vi "Configure Dialog.vi"(8 "error in (no error)":errorcluster, 11 "Configure Trigger Coupling Msg.lvclass":refnum<class "Configure Trigger Coupling Msg.lvclass">) -> (0 "error out":errorcluster, 2 "Ok?":bool, 3 "Configure Trigger Coupling Msg.lvclass":refnum<class "Configure Trigger Coupling Msg.lvclass">)   [LabVIEW 2014, in "CS++Scope.lvlib" / "Configure Trigger Coupling Msg.lvclass"]
uses:
  Configure Trigger Coupling Msg.lvclass
  Configure Trigger Coupling Msg.lvclass/Configure Trigger Coupling Msg.ctl
panel:
  in  "trigger coupling (DC)":i32
  in  "Cancel Button":bool
  in  "OK Button":bool
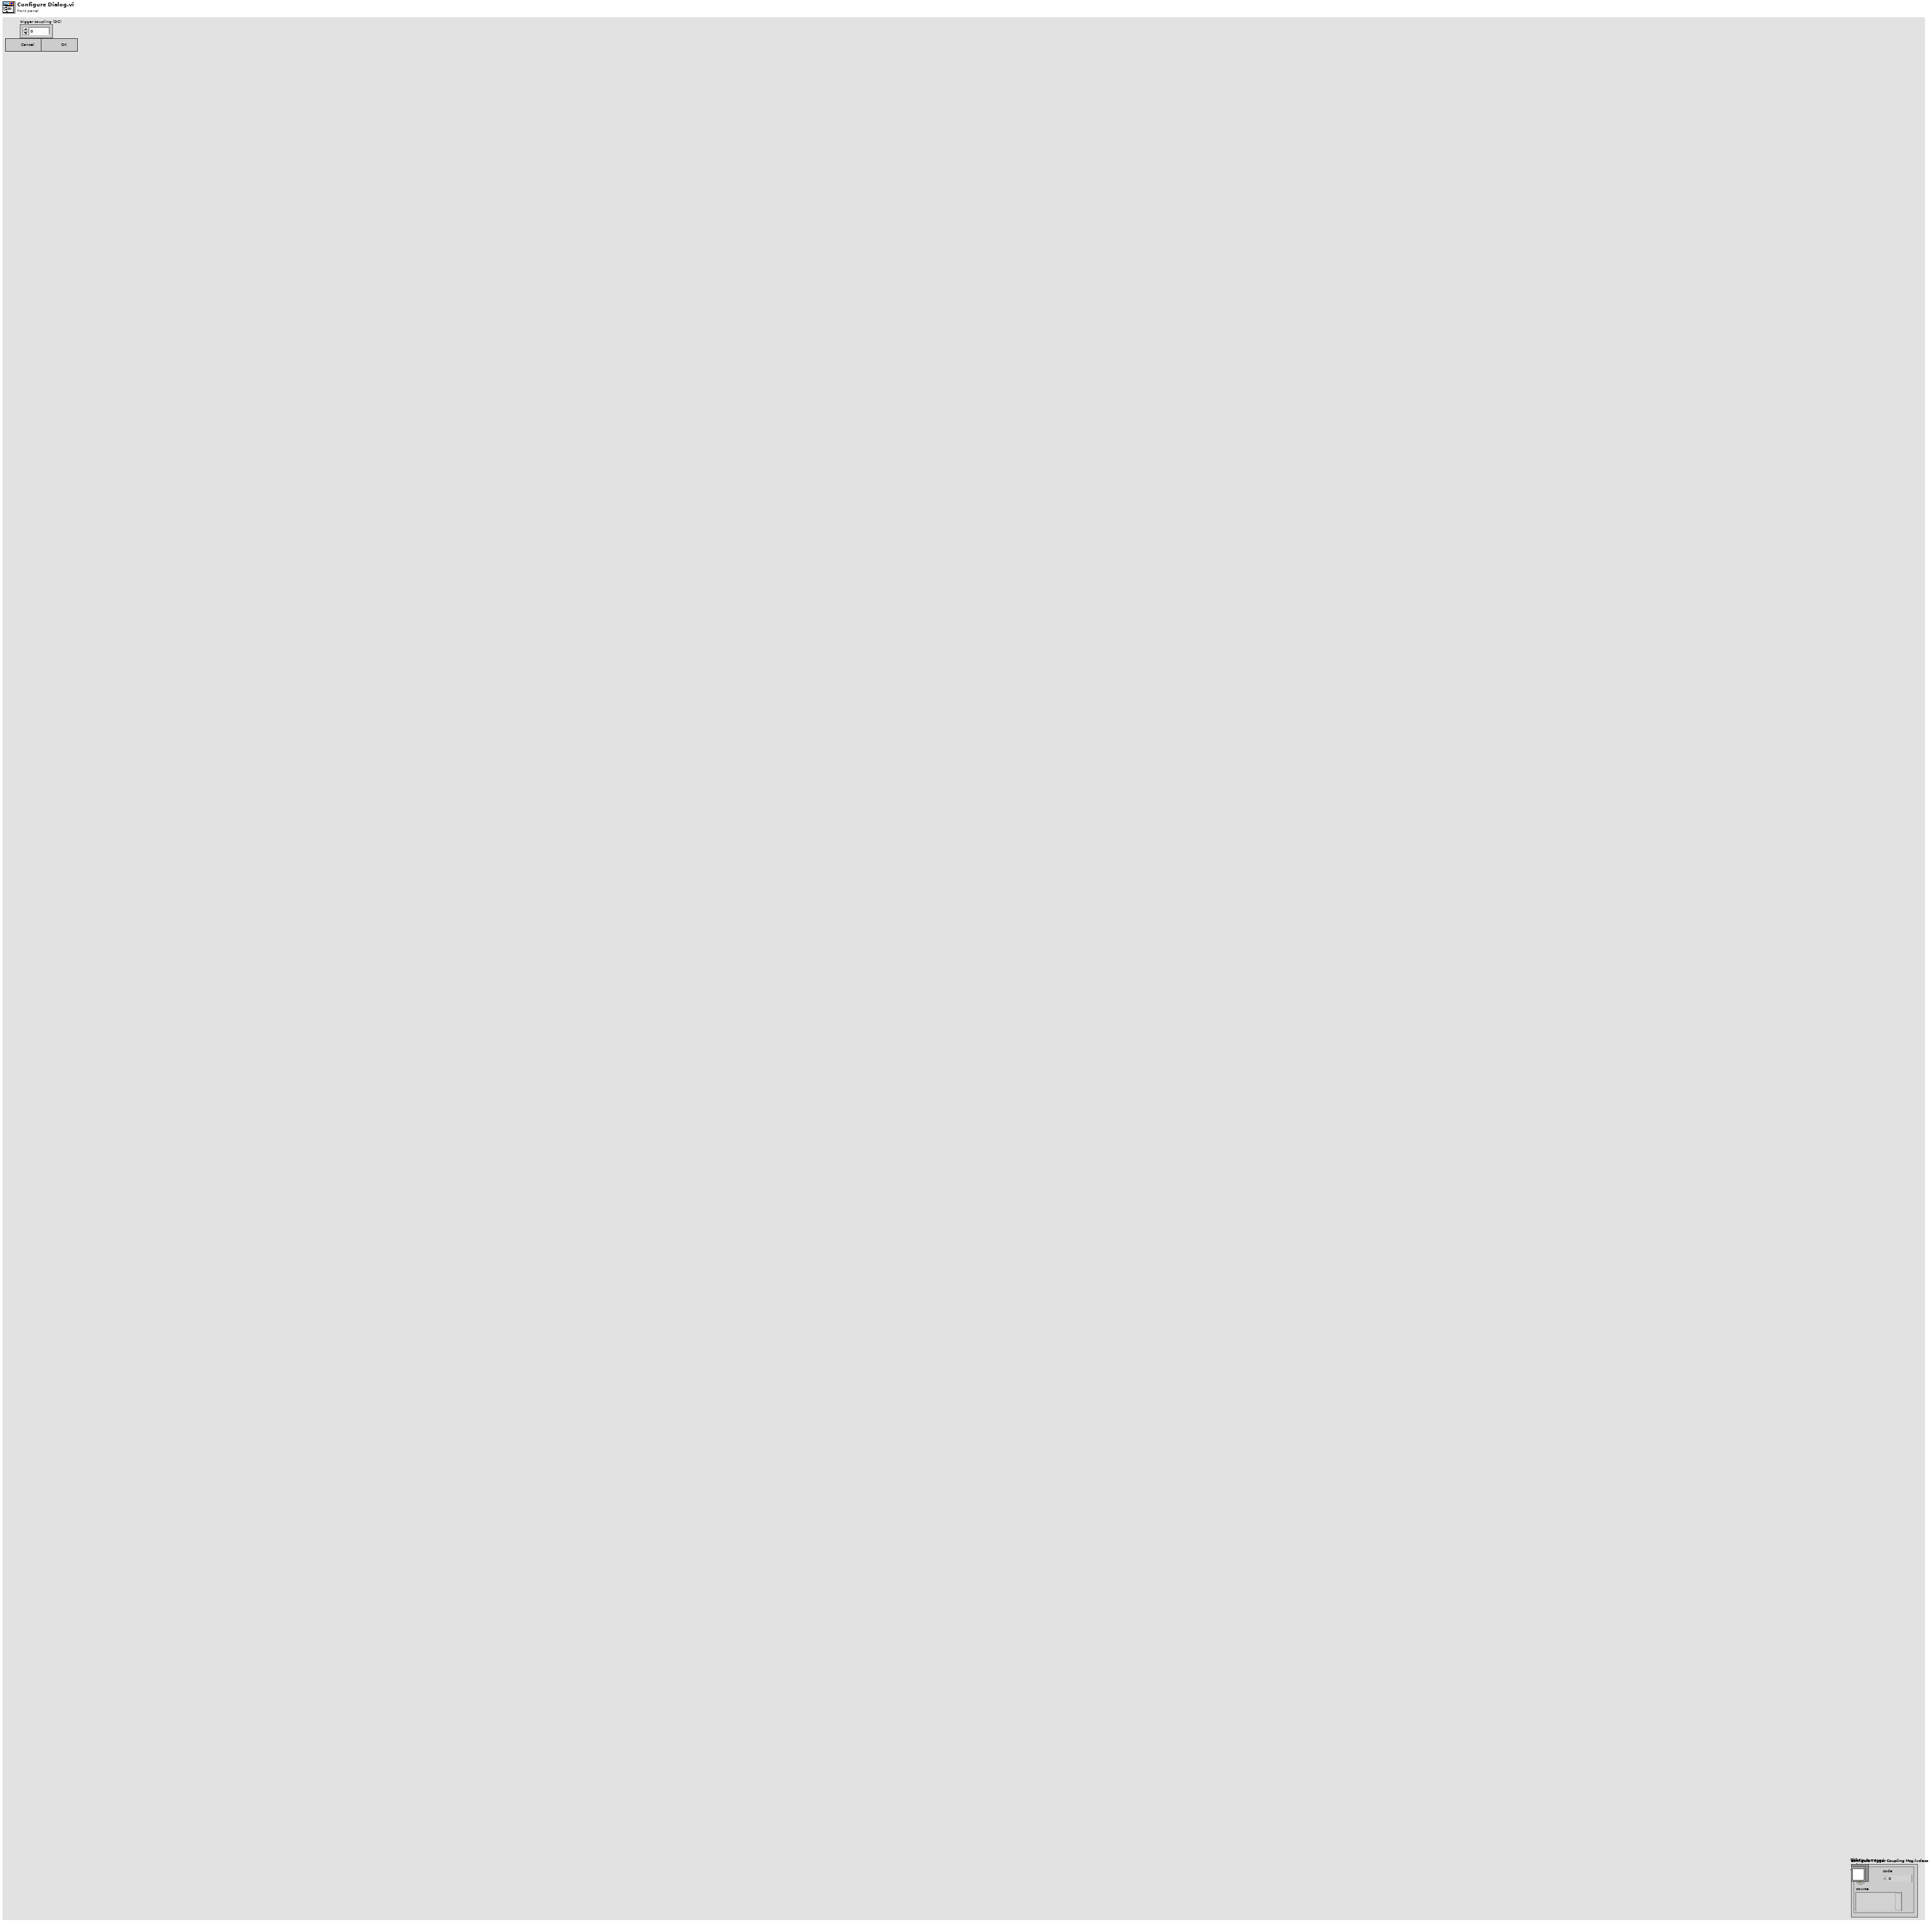
[diagram p1: front panel]
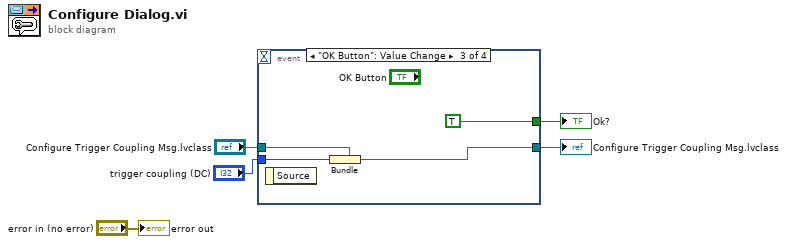
[diagram p0: block diagram]
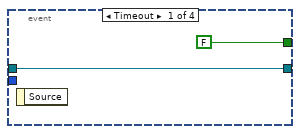
[diagram p2: hidden frame]
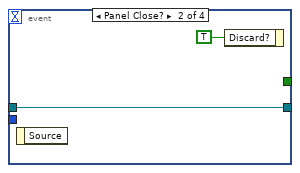
[diagram p3: hidden frame]
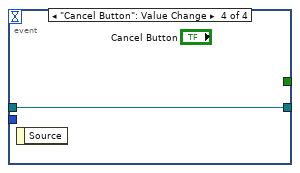
[diagram p4: hidden frame]
diagram:
  n1 = event shown="[2] \"OK Button\": Value Change" {
    selector: _ -> [_ _ _ _]
    dyn-events: _ -> [_ _ _ _]
    timeout: _ -> [_ _ _ _]
    tunnel: [w6 w8 w11 w14] -> w3
    tunnel: "Configure Trigger Coupling Msg.lvclass" -> [w6 w8 w13 w14]
    tunnel: [FALSE _ TRUE _] -> w4
    tunnel: "trigger coupling (DC)" -> [_ _ w10 _]
    event Timeout {
      n2 = event-data() -> ()  [unwired: 1 in, 1 out]
    }
    event Panel Close? {
      n3 = event-data() -> ()  [unwired: 1 in, 1 out]
      n4 = event-data ("Event Filter Node")("Discard?"=TRUE) -> ()  [unwired: 1 in, 1 out]
    }
    event "OK Button": Value Change {
      n5 = event-data() -> ()  [unwired: 1 in, 1 out]
      n6 = Bundle ("Main-Bundler")(cluster=w13, w10) -> (w11:refnum<class "Configure Trigger Coupling Msg.lvclass">)
    }
    event "Cancel Button": Value Change {
      n7 = event-data() -> ()  [unwired: 1 in, 1 out]
    }
  }
  "Ok?" <- w4
  "Configure Trigger Coupling Msg.lvclass" <- w3
  "error out" <- "error in (no error)"
